vi "SVPO Limit Testing (1 Ch) (SGL Waveform).vi"(7 "reset? (F)":bool, 9 "lower limit":sgl=-inf format="%.2f", 10 "upper limit":sgl=inf format="%.2f", 11 "signal in":waveform(sgl)) -> (1 "lower limit clearance":sgl format="%.6f", 2 "upper limit clearance":sgl format="%.6f", 3 "test passed?":bool, 5 "timestamps":T1 {"last failure" format="%<%.6X\n%x>T"; "first failure" format="%<%.6X\n%x>T"; "reset" format="%<%.6X\n%x>T"})   [LabVIEW 2017, in "SoundVib_LimitTest.lvlib"]
doc: "Performs limit testing on single-precision waveforms, single-precision scaled arrays, or double-precision scalar measurements. You can specify an upper and lower boundary of the envelope to define a pass range. This VI uses the defined pass range to test the input signal. VI outputs apply to all the tests since the last VI reset. Use this VI on embedded targets that have limited computational resources. Wire data to the <B>value in</B> input to determine the polymorphic instance to use or manually select the instance."
uses:
  <vilib>/addons/Sound and Vibration/svt_Limit Test/SoundVib_LimitTest.lvlib
  <vilib>/addons/Sound and Vibration/svt_Limit Test/SVPO Limit Testing (1 Ch) (SGL Array) with IC.vi
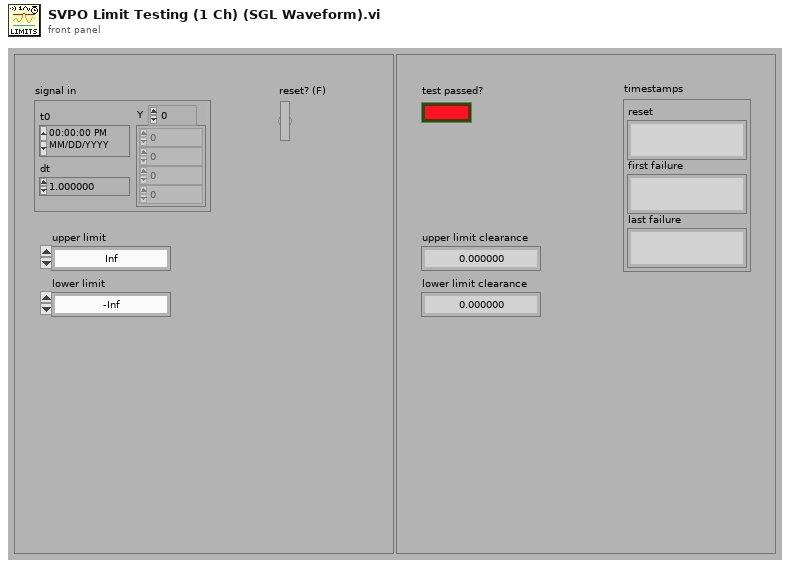
[diagram p1: front panel]
types:
  T1 = cluster{"reset":timestamp, "first failure":timestamp, "last failure":timestamp}
  T2 = typedef "svc_Waveform Limit State.ctl" = cluster{"timestamps":cluster{"reset":timestamp, "first failure":timestamp, "last failure":timestamp}, "limit state":T3}
  T3 = typedef "svc_SGL Limit State.ctl" = cluster{"upper limit clearance":sgl, "lower limit clearance":sgl, "test passed?":bool, "block passed?":bool}
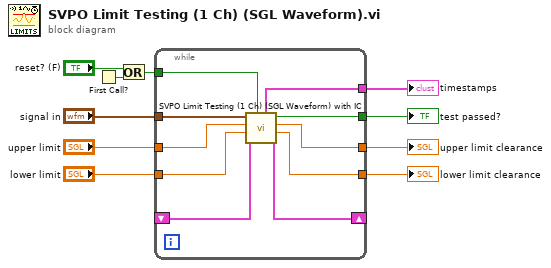
[diagram p0: block diagram]
diagram:
  n1 = First Call?() -> (First Call?: T/F=w6:bool)
  n2 = Or(x="reset? (F)", y=w6) -> (x .or. y?=w7:bool)
  n3 = while {
    tunnel: "signal in" -> [w20]
    tunnel: "upper limit" -> [w16]
    tunnel: "lower limit" -> [w15]
    tunnel: w7 -> [w18]
    tunnel: [w19] -> w4
    tunnel: [w17] -> w3
    tunnel: [w14] -> w2
    tunnel: [w13] -> w1
    shift-right: [w12] -> _
    shift-left: _ -> [w11]
    stop <- TRUE stop-if-true
    n4 = call <vilib>:"SVPO Limit Testing (1 Ch) (SGL Waveform) with IC.vi"("reset? (F)"=w18, "initial conditions"=w11, "lower limit"=w15, "upper limit"=w16, "signal in"=w20) -> ("final conditions"=w12:T2, "lower limit clearance"=w13:sgl, "upper limit clearance"=w14:sgl, "test passed?"=w19:bool, "timestamps"=w17:T1)  [unwired: 2 in]
  }
  "test passed?" <- w4
  "upper limit clearance" <- w2
  "lower limit clearance" <- w1
  "timestamps" <- w3
